vi "仁科测控RS-KTC-N01空调控制器.vi"() -> ()   [LabVIEW 2016, in "环境动力监测库.lvlib" / "空调库.lvlib"]
panel:
  out "Port":string
  out "IP":string
  out "x+1":u32
  in  "校时":bool
  out "仪器时间":timestamp format="%<%Y/%m/%d %H:%M:%S>T"
  out "运行状态":T1
  out "传感器状态输出":T2
  out "温湿度解析":cluster{"湿度":dbl, "温度":dbl}
  out "告警状态":T3
  in  "解除告警":bool
  out "串口":string
  in  "查看型号":bool
  in  "重开串口":bool
  in  "设定参数":bool
  in  "遥控":bool
  out "通讯":bool=TRUE
  # "A"
  # "A"
  # "℃"
  # "%"
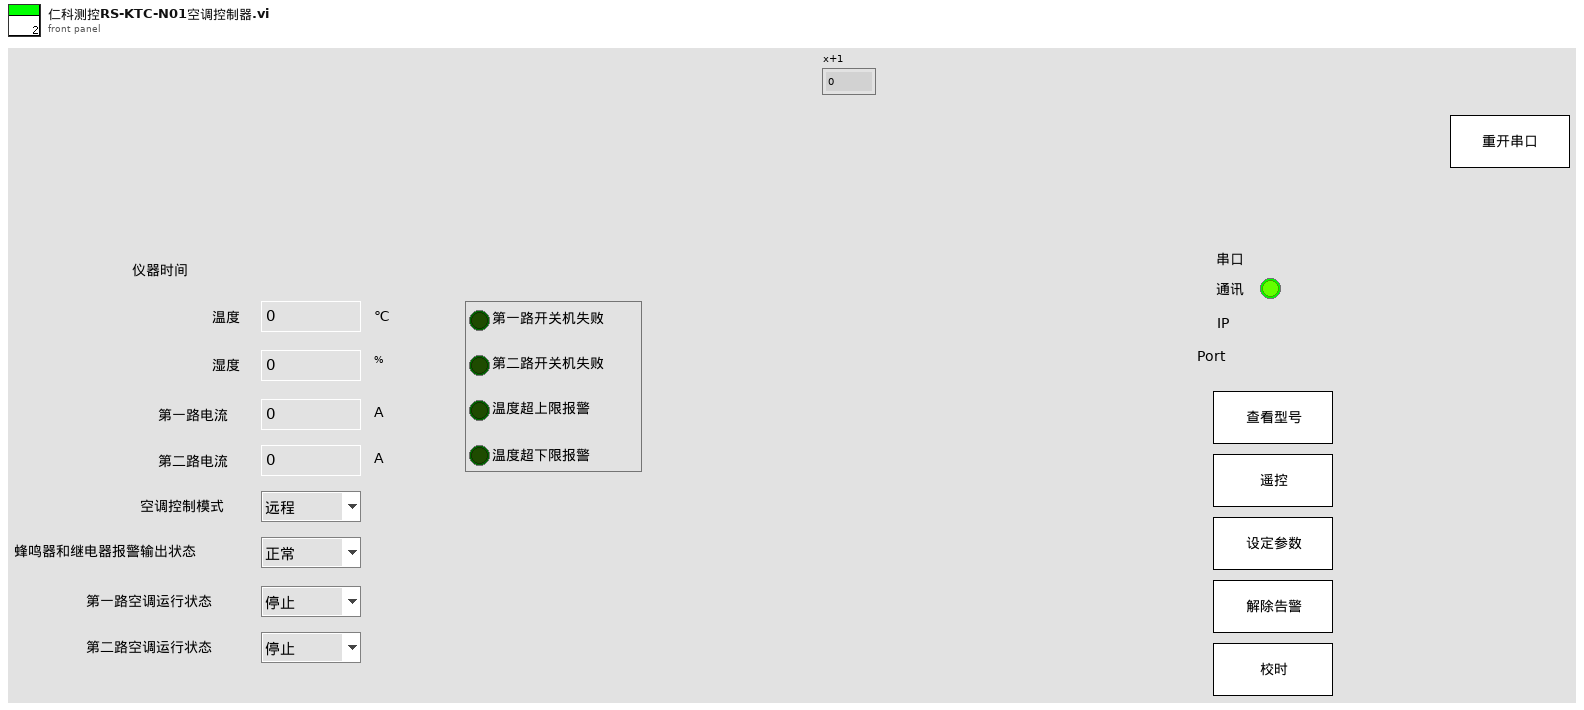
[diagram p1: front panel]
types:
  T1 = cluster{"第一路空调运行状态":enum16{"停止", "制冷", "制热", "未知"}, "第二路空调运行状态":enum16{"停止", "制冷", "制热", "未知"}}
  T2 = cluster{"第一路电流":dbl, "第二路电流":dbl, "空调控制模式":enum16{"远程", "自动"}, "蜂鸣器和继电器报警输出状态":enum16{"正常", "报警"}, "秒数高16位":u16, "秒数低16位":u16}
  T3 = cluster{"第一路开关机失败":bool, "第二路开关机失败":bool, "温度超上限报警":bool, "温度超下限报警":bool}
  T4 = enum32{"Bad", "Idle", "Run top level", "Running"}
  T5 = enum16{"open", "read", "write single", "write", "close"}
  T6 = cluster{"型号选择":enum16{"黑盾", "英维克", "仁科测控RS-KTC-N01"}, "MB session in":refnum<class "MB_Master.lvclass">, "英维克空调寄存器":u16[], "通讯状态":bool, "PORT":string, "IP":string, "Slave ID ":u8, "Serial Config":cluster{"baud rate (bps)":u32, "stop bits":u16, "parity":u16, "flow control":u16, "timeout":u32, "retries":i32}, "VISA Resource":refnum<visa-resource-name>, "MB通信方式选择":enum16{"串口", "TCP"}, "系统参数":cluster{"空调开启点":u16, "空调灵敏点":u16, "加热开启点":u16, "加热灵敏度":u16, "高温告警点":u16, "低温告警点":u16}}
  T7 = cluster{"漏水监测输出":cluster{"漏水监测告警":bool, "告警内容":string}, "门禁监测输出":cluster{"门禁监测告警":bool, "告警内容":string}, "门禁监测输出2":cluster{"门禁监测告警":bool, "告警内容":string}, "温湿度监测输出":cluster{"温湿度监测告警":bool, "告警内容":string}, "烟雾监测输出":cluster{"烟雾监测告警":bool, "告警内容":string}, "空调监测输出":cluster{"空调监测告警":bool, "告警内容":string}, "自动重合闸输出":cluster{"自动重合闸告警":bool, "告警内容":string}, "红外入侵输出":cluster{"红外入侵告警":bool, "告警内容":string}, "振动输出":cluster{"振动告警":bool, "告警内容":string}, "UPS输出":cluster{"UPS告警":bool, "告警内容":string}, "蓄电池输出":cluster{"蓄电池告警":bool, "告警内容":string}, "蓄电池输出2":cluster{"蓄电池告警":bool, "告警内容":string}, "GPS输出":cluster{"定位告警":bool, "告警内容":string}, "北斗输出":cluster{"定位告警":bool, "告警内容":string}, "气象输出":cluster{"气象告警":bool, "告警内容":string}, "废液输出":cluster{"废液告警":bool, "告警内容":string}, "废液输出2":cluster{"废液告警":bool, "告警内容":string}}
  T8 = cluster{"温湿度解析":cluster{"湿度":dbl, "温度":dbl}, "传感器状态输出":cluster{"第一路电流A":u16, "第二路电流A":u16, "空调控制模式":enum16{"远程", "自动"}, "蜂鸣器和继电器报警输出状态":enum16{"正常", "报警"}, "秒数高16位":u16, "秒数低16位":u16}, "告警状态":cluster{"第一路开关机失败":bool, "第二路开关机失败":bool, "温度超上限报警":bool, "温度超下限报警":bool}, "运行状态":cluster{"第一路空调运行状态":enum16{"停止", "制冷", "制热", "未知"}, "第二路空调运行状态":enum16{"停止", "制冷", "制热", "未知"}}}
  T9 = cluster{"第一路电流A":u16, "第二路电流A":u16, "空调控制模式":enum16{"远程", "自动"}, "蜂鸣器和继电器报警输出状态":enum16{"正常", "报警"}, "秒数高16位":u16, "秒数低16位":u16}
  T10 = cluster{"温湿度":cluster{"状态":bool, "温度:":sgl, "湿度:":sgl, "详情  ":bool}, "空调":cluster{"状态":bool, "机柜温度:":sgl, "压缩机:":enum16{"停止", "运行"}, "电加热:":enum16{"停止", "运行"}, "详情  ":bool}, "排气扇":cluster{"排气扇":bool, "详情  ":bool}, "冰箱":cluster{"冰箱":bool, "详情  ":bool}}
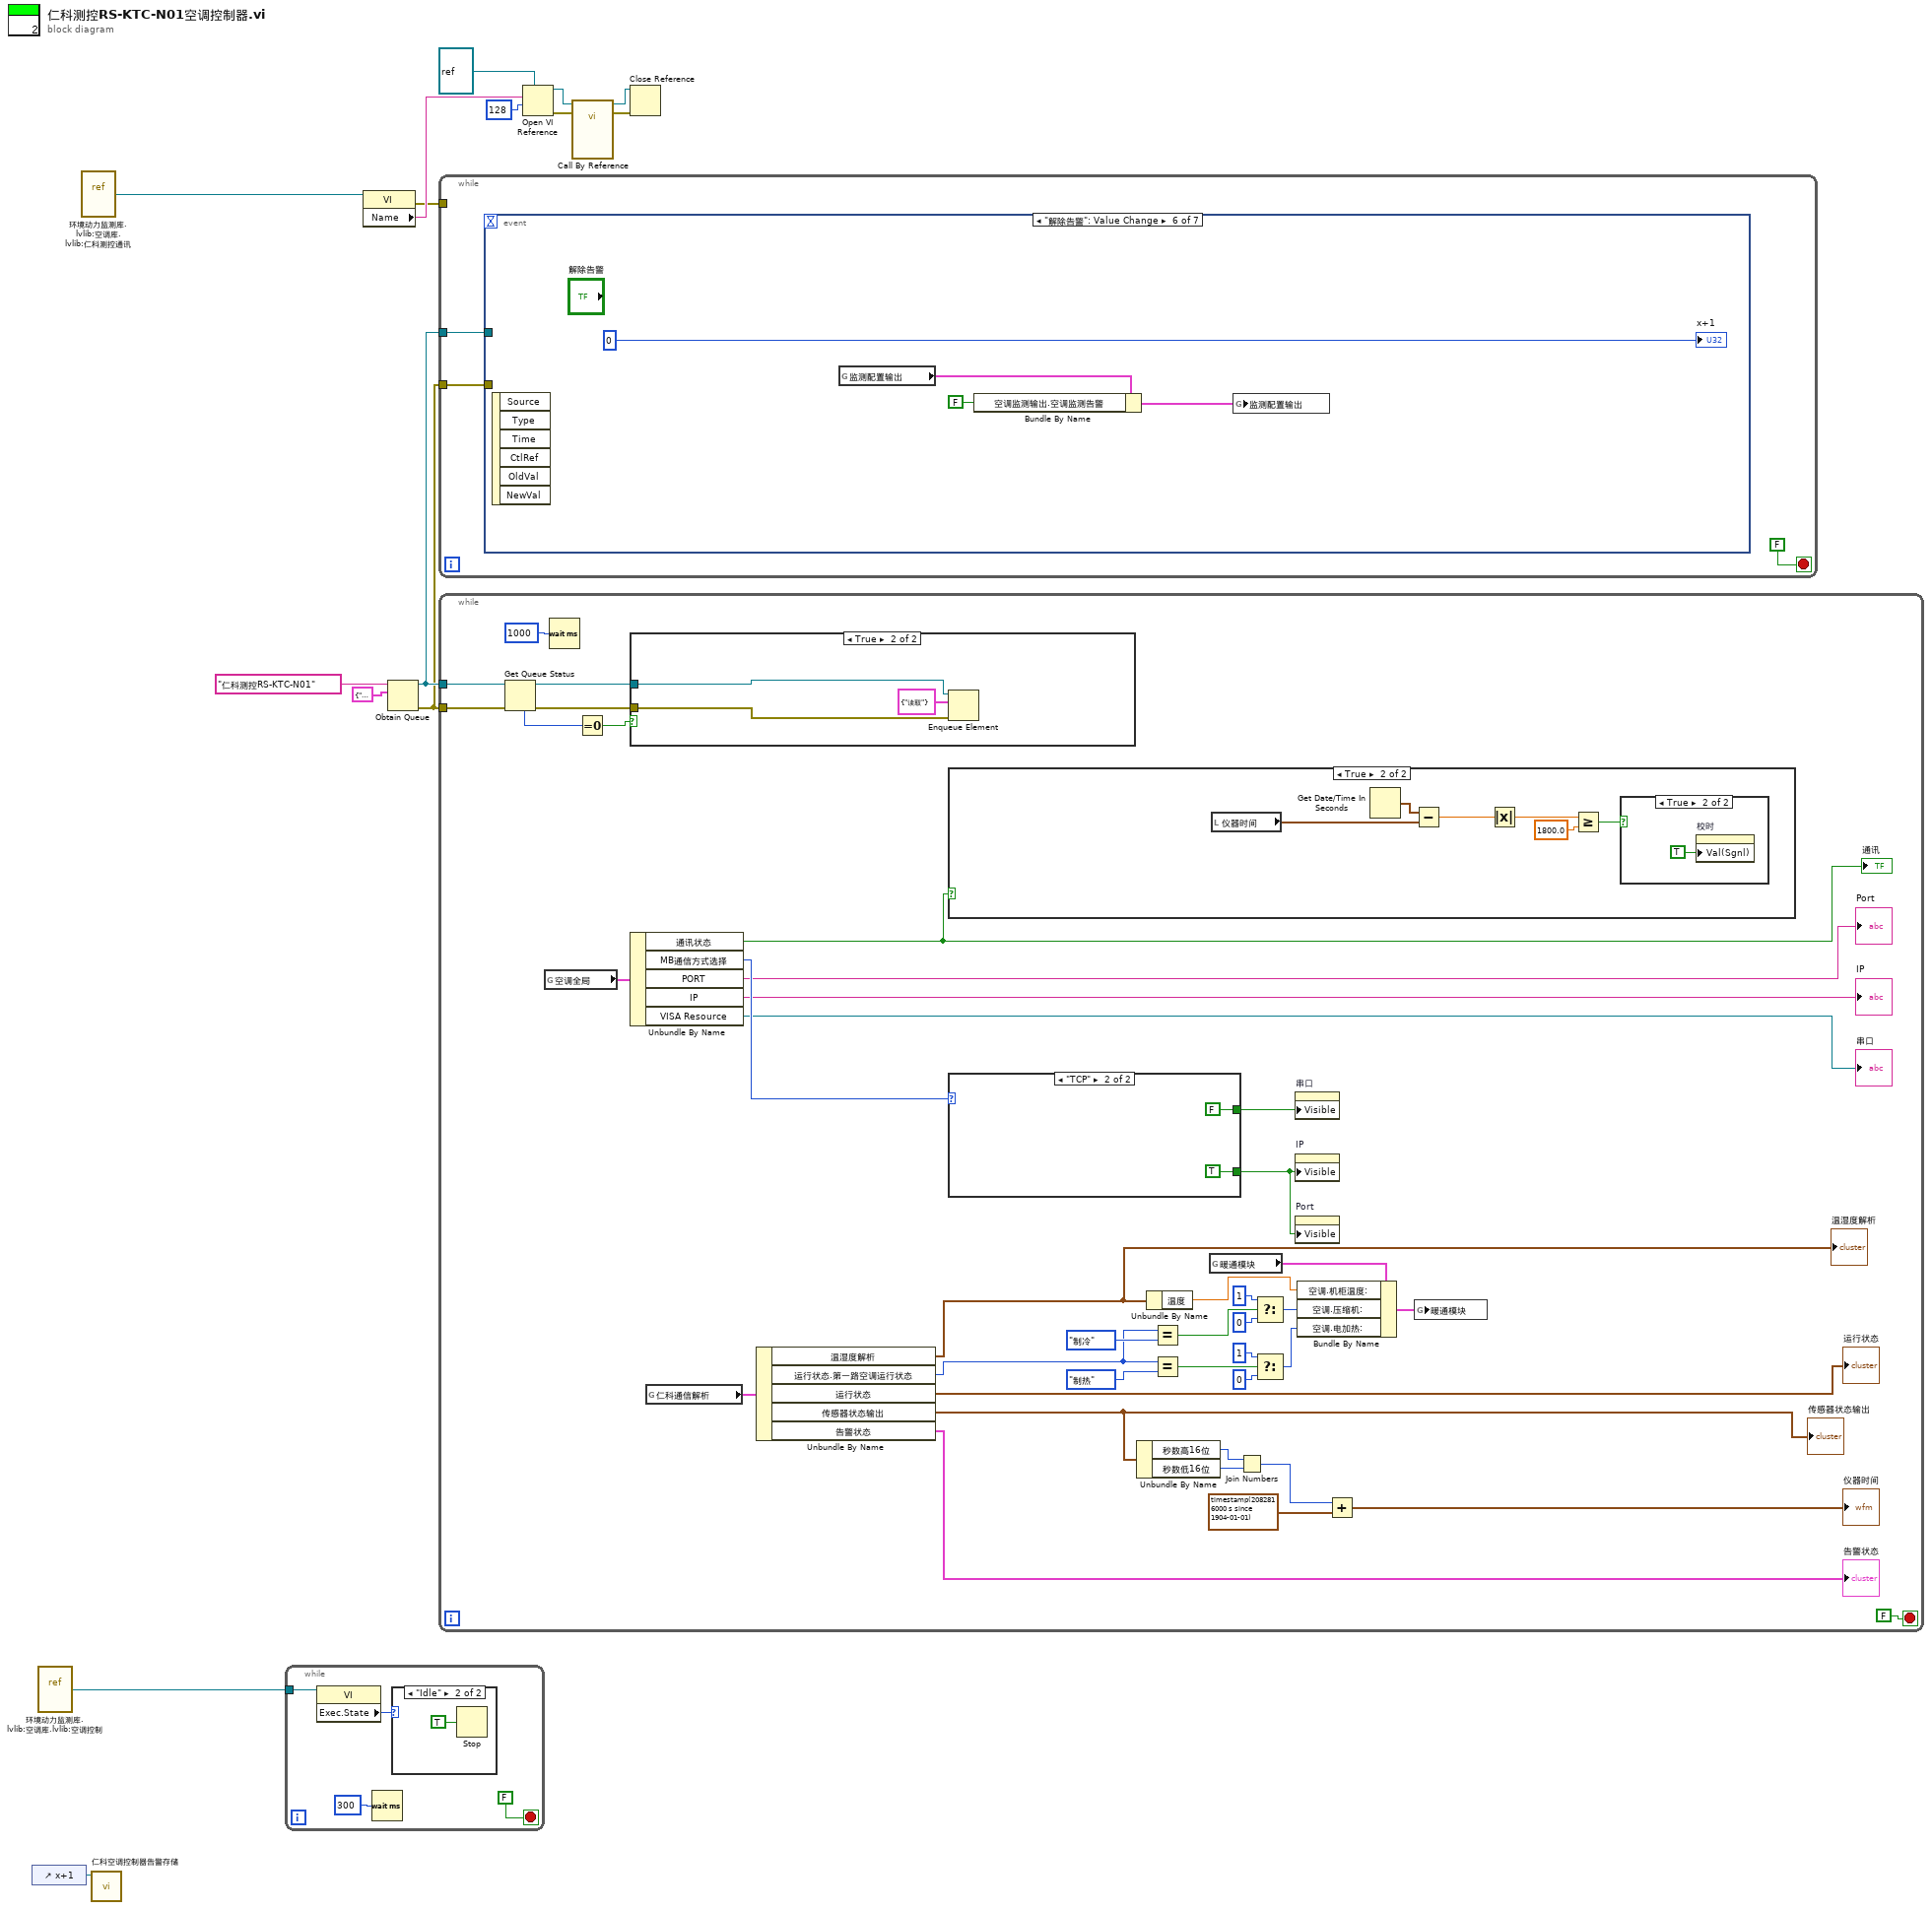
[diagram p0: block diagram]
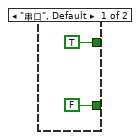
[diagram p3: hidden frame]
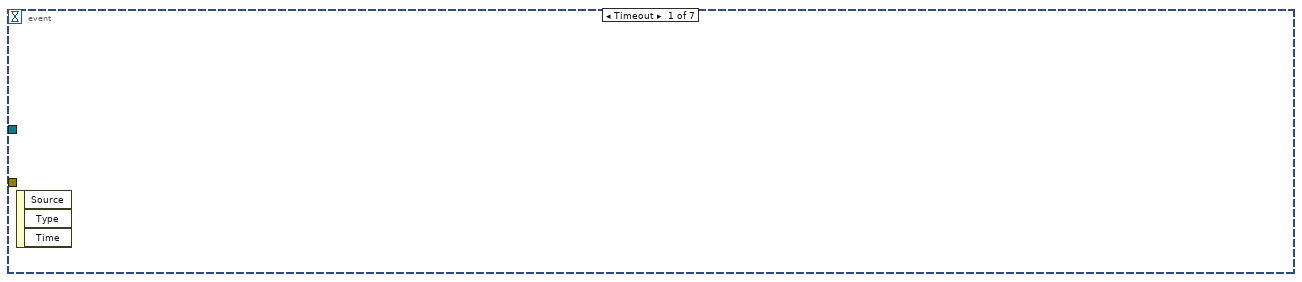
[diagram p7: hidden frame]
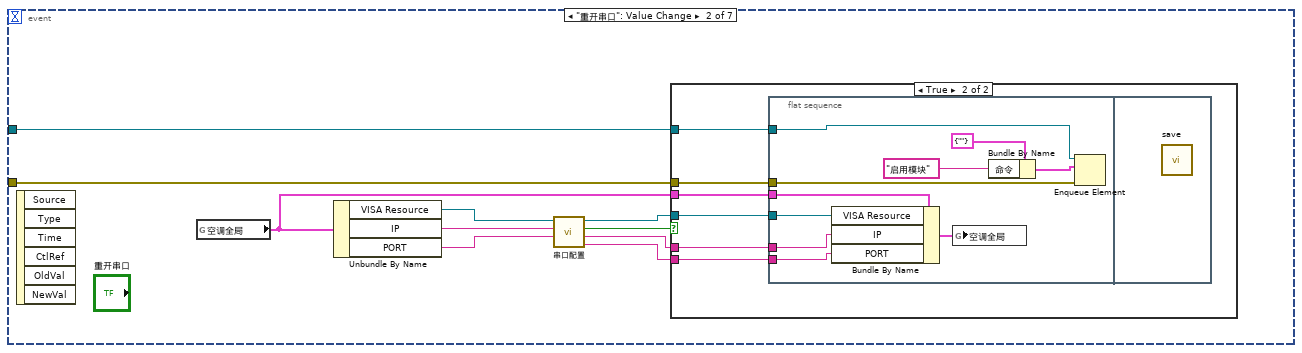
[diagram p8: hidden frame]
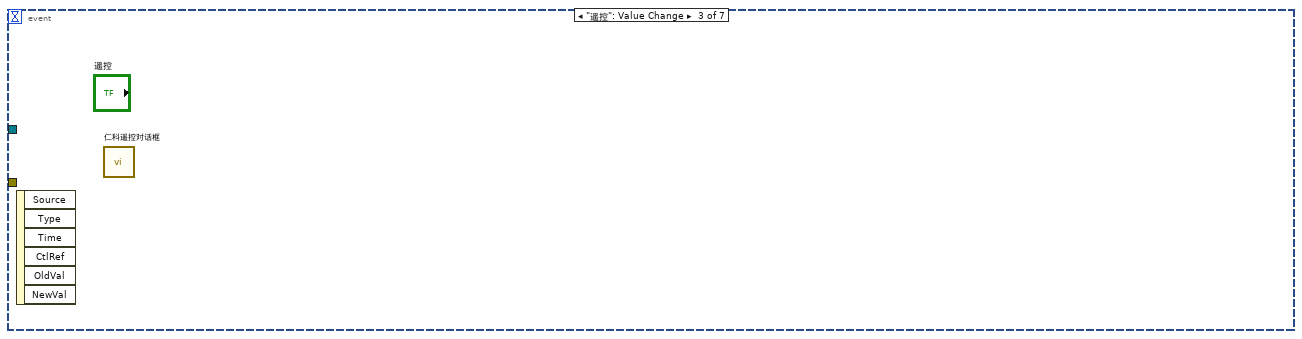
[diagram p10: hidden frame]
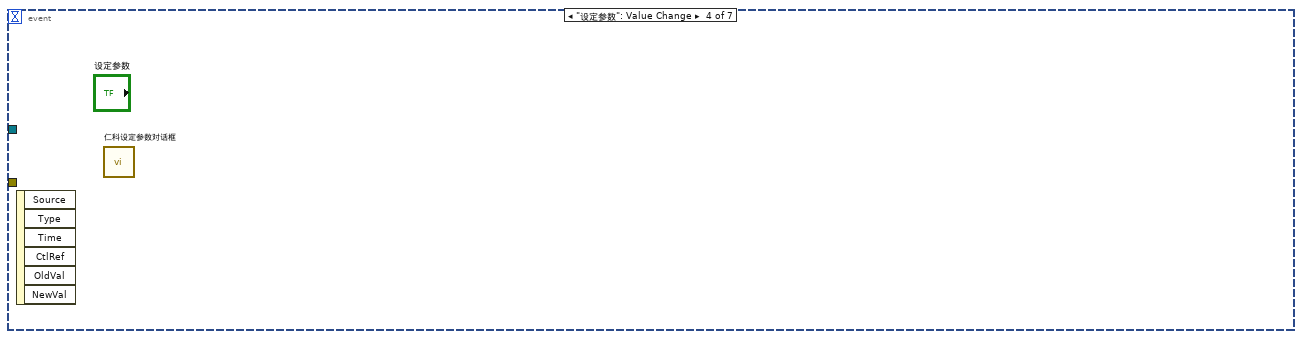
[diagram p11: hidden frame]
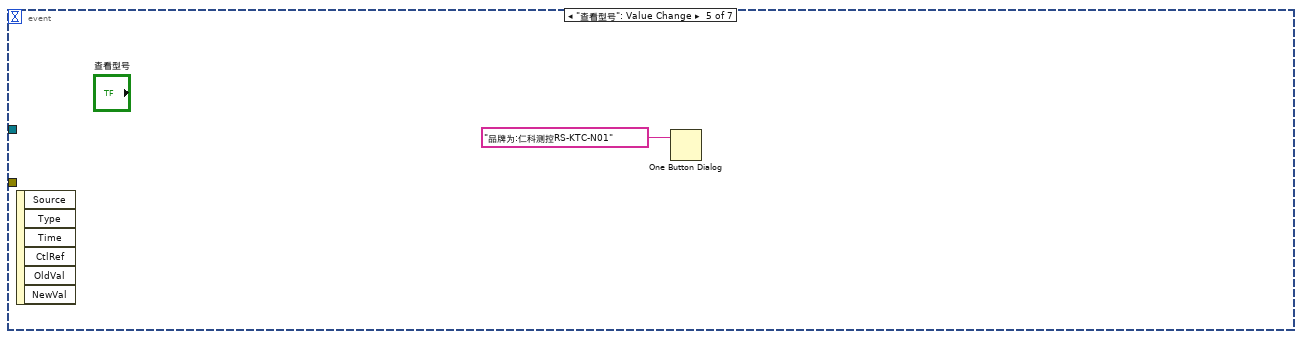
[diagram p12: hidden frame]
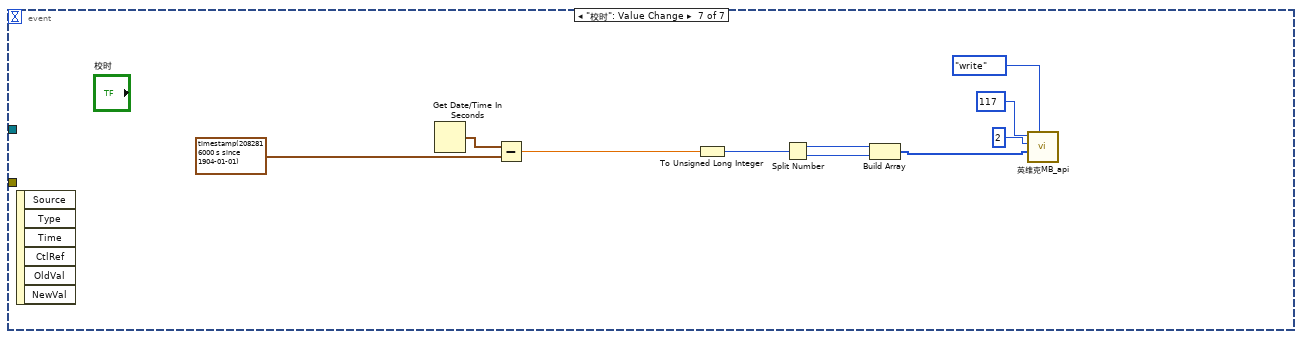
[diagram p13: hidden frame]
diagram:
  n1 = control-ref of="x+1"() -> (w1:refnum<vi>)
  n2 = vi-ref "环境动力监测库.lvlib:空调库.lvlib:空调控制.vi"() -> (w2:refnum<vi>)
  n3 = vi-ref "环境动力监测库.lvlib:空调库.lvlib:仁科测控通讯.vi"() -> (w8:refnum<vi>)
  n4 = call "仁科空调控制器告警存储.vi"("x+1"=w1) -> ()  [unwired: 11 in]
  n5 = while {
    tunnel: w2 -> [w19]
    stop <- FALSE stop-if-true
    n6 = property class="VI"(reference=w19) -> ("Exec.State"=w18:T4)  [unwired: 1 in, 2 out]
    n7 = Wait (ms)(milliseconds to wait=u32 300 ("等待时间（毫秒）")) -> ()  [unwired: 1 out]
    n8 = case shown="\"Idle\"" w18 {
      frame "Bad", Default {
      }
      frame "Idle" {
        n9 = Stop(stop? (T)=TRUE ("停止？(T)")) -> ()
      }
    }
  }
  n10 = property class="VI"(reference=w8) -> (error out=w3:errorcluster, "Name"=w9:string)  [unwired: 1 in, 1 out]
  n11 = Obtain Queue(name (unnamed)="仁科测控RS-KTC-N01" ("名称（未命名）"), element data type=cluster{"命令":string} {"命令"="启用模块"} ("元素")) -> (queue out=w5:refnum<queue>, error out=w4:errorcluster)  [unwired: 3 in, 1 out]
  n12 = while {
    tunnel: w5 -> [w22]
    tunnel: w4 -> [w21]
    tunnel: w3 -> [_]
    stop <- FALSE stop-if-true
    n13 = event shown="[5] \"解除告警\": Value Change" {
      selector: _ -> [_ _ _ _ _ _ _]
      dyn-events: _ -> [_ _ _ _ _ _ _]
      timeout: _ -> [_ _ _ _ _ _ _]
      tunnel: w22 -> [_ w29 _ _ _ _ _]
      tunnel: w21 -> [_ w28 _ _ _ _ _]
      event Timeout {
        n14 = event-data() -> ()  [unwired: 1 in, 3 out]
      }
      event "重开串口": Value Change {
        n15 = event-data() -> ()  [unwired: 1 in, 6 out]
        n16 = global read "断电保存全局变量.vi" "空调全局"() -> (w24:T6)
        n17 = Unbundle By Name(w24) -> ("VISA Resource"=w25:refnum<visa-resource-name>, "IP"=w27:string, "PORT"=w26:string)
        n18 = call "串口配置.vi"("PORT"=w26, "IP"=w27, "请选择串口:"=w25) -> ("PORT 2"=w30:string, "IP 2"=w31:string, "确认 2"=w32:bool, "VISA资源名称 2"=w33:refnum<visa-resource-name>)  [unwired: 5 in]
        n19 = case shown="True" w32 {
          tunnel: w33 -> [_ w37]
          tunnel: w29 -> [_ w39]
          tunnel: w28 -> [_ w38]
          tunnel: w31 -> [_ w36]
          tunnel: w30 -> [_ w35]
          tunnel: w24 -> [_ w34]
          frame False {
          }
          frame True {
            n20 = flat-sequence {
              tunnel: w39 -> [w46]
              tunnel: w38 -> [w45]
              tunnel: w37 -> [w43]
              tunnel: w36 -> [w42]
              tunnel: w35 -> [w41]
              tunnel: w34 -> [w44]
              frame #0 {
                n21 = Bundle By Name(cluster=w44, "VISA Resource"=w43, "IP"=w42, "PORT"=w41) -> (w40:T6)
                n22 = global write "断电保存全局变量.vi" "空调全局"(w40) -> ()
                n23 = Bundle By Name(cluster=cluster{"命令":string} {"命令"=""} ("元素"), "命令"="启用模块" ("名称（未命名）")) -> (w47:cluster{"命令":string})
                n24 = Enqueue Element(queue=w46, element=w47, error in (no error)=w45) -> ()  [unwired: 1 in, 3 out]
              }
              frame #1 {
                n25 = call "save.vi"() -> ()  [unwired: 11 in, 1 out]
              }
            }
          }
        }
      }
      event "遥控": Value Change {
        n26 = event-data() -> ()  [unwired: 1 in, 6 out]
        n27 = call "仁科遥控对话框.vi"() -> ()  [unwired: 12 in]
      }
      event "设定参数": Value Change {
        n28 = event-data() -> ()  [unwired: 1 in, 6 out]
        n29 = call "仁科设定参数对话框.vi"() -> ()  [unwired: 12 in]
      }
      event "查看型号": Value Change {
        n30 = event-data() -> ()  [unwired: 1 in, 6 out]
        n31 = One Button Dialog(message="品牌为:仁科测控RS-KTC-N01" ("消息")) -> ()  [unwired: 1 in, 1 out]
      }
      event "解除告警": Value Change {
        n32 = event-data() -> ()  [unwired: 1 in, 6 out]
        n33 = global read "内部交互全局变量.vi" "监测配置输出"() -> (w52:T7)
        n34 = Bundle By Name(cluster=w52, "空调监测输出.空调监测告警"=FALSE) -> (w51:T7)
        n35 = global write "内部交互全局变量.vi" "监测配置输出"(w51) -> ()
        "x+1" <- u32 0 ("x+1")
      }
      event "校时": Value Change {
        n36 = event-data() -> ()  [unwired: 1 in, 6 out]
        n37 = Get Date/Time In Seconds() -> (seconds since 1Jan1904=w56:timestamp)
        n38 = Subtract(x=w56, y=timestamp(2082816000 s since 1904-01-01) ("当前时间")) -> (x-y=w60:dbl)
        n39 = To Unsigned Long Integer(number=w60) -> (unsigned 32bit integer=w59:u32)
        n40 = Split Number(x=w59) -> (hi(x)=w58:u16, lo(x)=w57:u16)
        n41 = Build Array(w58, w57) -> (w61:u16[])
        n42 = call "英维克MB_api.vi"("STEP"=T5."write", "values"=w61, "quantity"=u16 2, "starting address"=u16 117) -> ()  [unwired: 5 in, 3 out]
      }
    }
  }
  n43 = while {
    tunnel: w5 -> [w103]
    tunnel: w4 -> [w102]
    stop <- FALSE stop-if-true
    n44 = Get Queue Status(queue=w103, error in (no error)=w102) -> (queue out=w100:refnum<queue>, error out=w99:errorcluster, # elements in queue=w104:i32)  [unwired: 1 in, 5 out]
    n45 = global read "断电保存全局变量.vi" "空调全局"() -> (w70:T6)
    n46 = Wait (ms)(milliseconds to wait=u32 1000 ("等待时间（毫秒）")) -> ()  [unwired: 1 out]
    n47 = Equal To 0?(x=w104) -> (x = 0?=w101:bool)
    n48 = case shown="True" w101 {
      tunnel: w100 -> [_ w118]
      tunnel: w99 -> [_ w117]
      frame False {
      }
      frame True {
        n49 = Enqueue Element(queue=w118, element=cluster{"命令":string} {"命令"="读取"} ("元素"), error in (no error)=w117) -> ()  [unwired: 1 in, 3 out]
      }
    }
    n50 = Unbundle By Name(w70) -> ("通讯状态"=w65:bool, "MB通信方式选择"=w69:enum16{"串口", "TCP"}, "PORT"=→"Port":string, "IP"=→"IP":string, "VISA Resource"=→"串口":refnum<visa-resource-name>)
    "通讯" <- w65
    n51 = global read "内部交互全局变量.vi" "仁科通信解析"() -> (w90:T8)
    n52 = Unbundle By Name(w90) -> ("温湿度解析"=w80:cluster{"湿度":dbl, "温度":dbl}, "运行状态.第一路空调运行状态"=w86:enum16{"停止", "制冷", "制热", "未知"}, "运行状态"=→"运行状态":T1, "传感器状态输出"=w78:T9, "告警状态"=→"告警状态":T3)
    "温湿度解析" <- w80
    "传感器状态输出" <- w78
    n53 = case shown="True" w65 {
      frame False {
      }
      frame True {
        n54 = local read "仪器时间"() -> (w114:timestamp)
        n55 = Get Date/Time In Seconds() -> (seconds since 1Jan1904=w109:timestamp)
        n56 = Subtract(x=w109, y=w114) -> (x-y=w113:dbl)
        n57 = Absolute Value(x=w113) -> (abs(x)=w112:dbl)
        n58 = Greater Or Equal?(x=w112, y=1800.0) -> (x >= y?=w110:bool)
        n59 = case shown="True" w110 {
          frame False {
          }
          frame True {
            n60 = property on="校时" class="Bool (strict)"("Val(Sgnl)"=TRUE ("值(信号)")) -> ()  [unwired: 2 in, 2 out]
          }
        }
      }
    }
    n61 = case shown="\"TCP\"" w69 {
      tunnel: [TRUE FALSE] -> w72
      tunnel: [FALSE TRUE] -> w71
      frame "串口", Default {
      }
      frame "TCP" {
      }
    }
    n62 = Unbundle By Name(w78) -> ("秒数高16位"=w77:u16, "秒数低16位"=w76:u16)
    n63 = Unbundle By Name(w80) -> ("温度"=w94:dbl)
    n64 = Equal?(x=w86, y=enum16{"停止", "制冷", "制热", "未知"}."制冷") -> (x = y?=w88:bool)
    n65 = Equal?(x=w86, y=enum16{"停止", "制冷", "制热", "未知"}."制热") -> (x = y?=w83:bool)
    n66 = global read "内部交互全局变量.vi" "暖通模块"() -> (w95:T10)
    n67 = Join Numbers(hi=w77, lo=w76) -> ((hi.lo)=w74:u32)
    n68 = Select(t=1, s=w88, f=0) -> (s? t:f=w91:i32)
    n69 = Select(t=1, s=w83, f=0) -> (s? t:f=w82:i32)
    n70 = property on="串口" class="Str"("Visible"=w72) -> ()  [unwired: 2 in, 2 out]
    n71 = property on="IP" class="Str"("Visible"=w71) -> ()  [unwired: 2 in, 2 out]
    n72 = property on="Port" class="Str"("Visible"=w71) -> ()  [unwired: 2 in, 2 out]
    n73 = Bundle By Name(cluster=w95, "空调.机柜温度:"=w94, "空调.压缩机:"=w91, "空调.电加热:"=w82) -> (w96:T10)
    n74 = Add(x=w74, y=timestamp(2082816000 s since 1904-01-01) ("当前时间")) -> (x+y=→"仪器时间":timestamp)
    n75 = global write "内部交互全局变量.vi" "暖通模块"(w96) -> ()
  }
  n76 = Open VI Reference(type specifier VI Refnum (for type only)=refnum<vi> refnum, vi path=w9, options=128 ("选项")) -> (vi reference=w11:refnum<vi>, error out=w13:errorcluster)  [unwired: 3 in]
  n77 = call-by-ref "?"(reference=w11, error in=w13) -> (reference out=w15:refnum<vi>, error out=w14:errorcluster)  [unwired: 12 in]
  n78 = Close Reference(reference=w15, error in (no error)=w14) -> ()  [unwired: 1 out]
